vi "widmo.vi"(11 "wykres":waveform(dbl)) -> (1 "wykres2":waveform(cdb), 2 "f_ps":cdb[](array[numeric]), 3 "ps":cdb[](array[numeric]), 4 "df":dbl, 5 "n2":dbl)   [LabVIEW 2025]
uses:
  <vilib>/Analysis/2dsp.llb/Real FFT.vi
  <vilib>/Analysis/NI_AALPro.lvlib
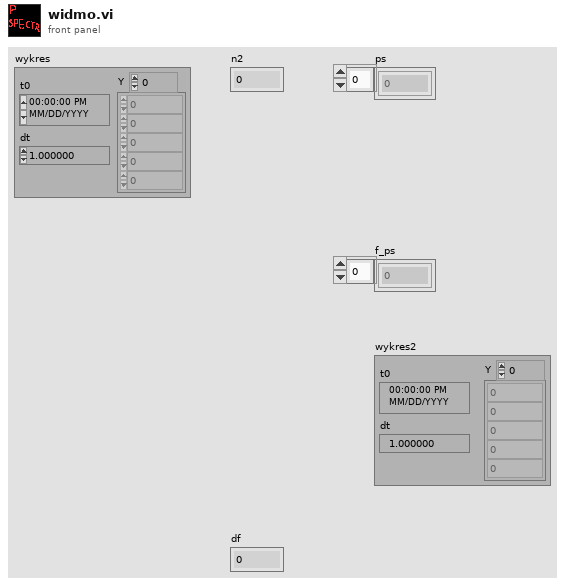
[diagram p1: front panel]
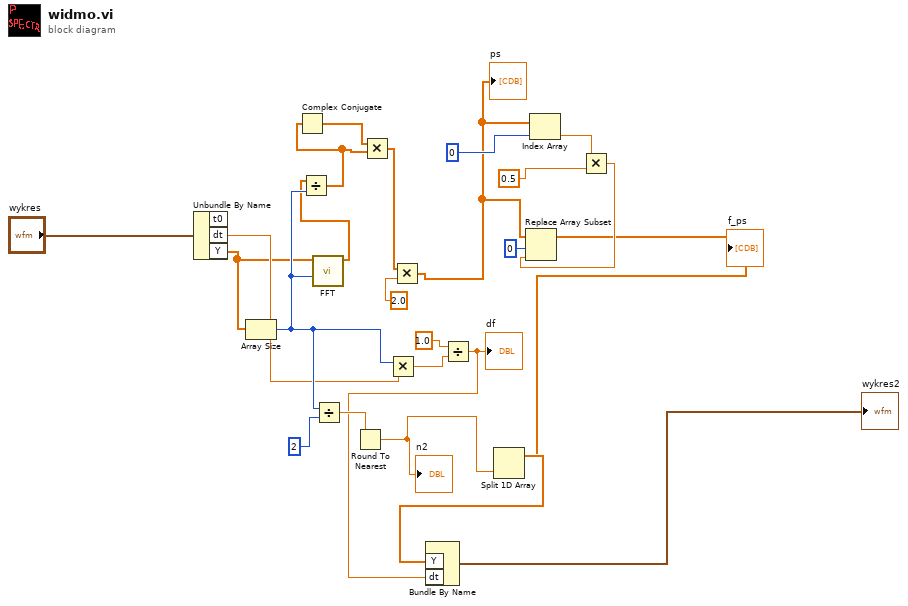
[diagram p0: block diagram]
diagram:
  n1 = Unbundle By Name("wykres") -> ("dt"=w9:dbl, "Y"=w2:dbl[])  [unwired: 1 out]
  n2 = Array Size(array=w2) -> (size(s)=w24:i32)
  n3 = call-poly <vilib>:"FFT.vi"("FFT size"=w24, "X"=w2) -> ("FFT {X}"=w23:cdb[])  [unwired: 8 in, 1 out]
  n4 = Divide(x=w23, y=w24) -> (x/y=w22:cdb[])
  n5 = Complex Conjugate(1:w22) -> (0:w20:cdb[])
  n6 = Divide(x=w24, y=2) -> (x/y=w15:dbl)
  n7 = Round To Nearest(number=w15) -> (nearest integer value=w8:dbl)
  "n2" <- w8
  n8 = Multiply(x=w20, y=w22) -> (x*y=w21:cdb[])
  n9 = Multiply(x=w24, y=w9) -> (x*y=w17:dbl)
  n10 = Multiply(x=w21, y=2.0) -> (x*y=w1:cdb[])
  "ps" <- w1
  n11 = Divide(x=1.0, y=w17) -> (x/y=w6:dbl)
  "df" <- w6
  n12 = Index Array(array=w1, index=0) -> (element=w12:cdb)
  n13 = Multiply(x=w12, y=0.5) -> (x*y=w11:cdb)
  n14 = Replace Array Subset(array=w1, new element=w11, index=0) -> (w3:cdb[])
  "f_ps" <- w3
  n15 = Split 1D Array(array=w3, index=w8) -> (first subarray=w4:cdb[])  [unwired: 1 out]
  n16 = Bundle By Name("Y"=w4, "dt"=w6) -> (→"wykres2":waveform(cdb))  [unwired: 1 in]
